vi "Adaptive graph scaling.vi"(7 "Reset buffer":bool, 8 "error in":errorcluster, 9 "Buffer length (points)":i32=10, 10 "Graph data":dbl[](array[numeric]), 11 "GraphChart":refnum<vi>) -> (0 "error out":errorcluster)   [LabVIEW 2017]
uses:
  <userlib>/_MGI/Numeric/Rounding/MGI Round to Decimal Place Enum.ctl
  <vilib>/Analysis/baseanly.llb/Mean (DBL).vi
  <userlib>/_MGI/Application Control/MGI Change Detector/MGI Change Detector (T).vi
  <vilib>/Analysis/NI_AALBase.lvlib
panel:
  # "Use the \"To more generic\" function outside this VI to\nallow using this VI with any type of graph."
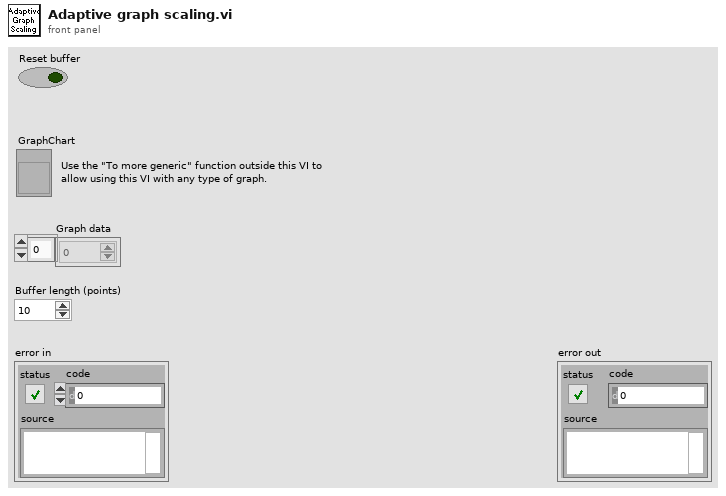
[diagram p1: front panel]
types:
  T1 = typedef "MGI Round to Decimal Place Enum.ctl" = enum16{"Round Nearest", "Round +Inf", "Round -Inf"}
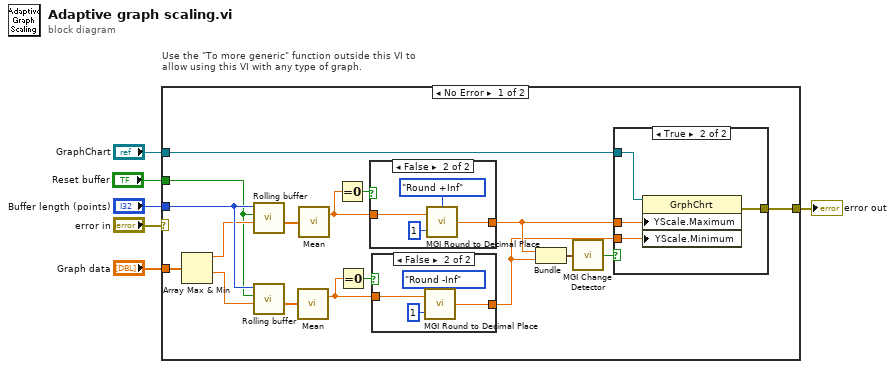
[diagram p0: block diagram]
diagram:
  # "Use the \"To more generic\" function outside this VI to\nallow using this VI with any type of graph."
  n1 = case shown="No Error" "error in" {
    selector: "error in" -> [_ w38]
    tunnel: "Buffer length (points)" -> [w23 _]
    tunnel: "Graph data" -> [w20 _]
    tunnel: "GraphChart" -> [w19 _]
    tunnel: [w8 w38] -> w2
    tunnel: "Reset buffer" -> [w7 _]
    frame No Error {
      n2 = Array Max & Min(array=w20) -> (max value=w22:dbl, min value=w21:dbl)  [unwired: 2 out]
      n3 = call "Rolling buffer.vi"("Value in"=w22, "Reset buffer"=w7, "Buffer length (points)"=w23) -> ("Rolling buffer"=w14:dbl[])  [unwired: 8 in]
      n4 = call "Rolling buffer.vi"("Value in"=w21, "Reset buffer"=w7, "Buffer length (points)"=w23) -> ("Rolling buffer"=w13:dbl[])  [unwired: 8 in]
      n5 = call-poly <vilib>:"Mean.vi"("X"=w13) -> ("mean"=w16:dbl)  [unwired: 1 out]
      n6 = call-poly <vilib>:"Mean.vi"("X"=w14) -> ("mean"=w18:dbl)  [unwired: 1 out]
      n7 = Equal To 0?(x=w18) -> (x = 0?=w17:bool)
      n8 = Equal To 0?(x=w16) -> (x = 0?=w15:bool)
      n9 = case shown="False" w17 {
        tunnel: w18 -> [w33 w35]
        tunnel: [w33 w34] -> w12
        frame True {
        }
        frame False {
          n10 = call <userlib>:"MGI Round to Decimal Place.vi"("Round (To Nearest)"=MGI_Round_to_Decimal_Place_Enum."Round +Inf", "Decimal Digits"=1, "Number"=w35) -> ("Rounded"=w34:dbl)
        }
      }
      n11 = case shown="False" w15 {
        tunnel: w16 -> [w28 w31]
        tunnel: [w28 w30] -> w11
        frame True {
        }
        frame False {
          n12 = call <userlib>:"MGI Round to Decimal Place.vi"("Round (To Nearest)"=MGI_Round_to_Decimal_Place_Enum."Round -Inf", "Decimal Digits"=1, "Number"=w31) -> ("Rounded"=w30:dbl)
        }
      }
      n13 = Bundle("Rounded"=w12, "Rounded"=w11) -> (w10:cluster{"Rounded":dbl, "Rounded":dbl})  [unwired: 1 in]
      n14 = call-poly <userlib>:"MGI Change Detector.vi"("Value"=w10) -> ("Changed?"=w9:bool)
      n15 = case shown="True" w9 {
        tunnel: w12 -> [_ w27]
        tunnel: w11 -> [_ w26]
        tunnel: w19 -> [_ w25]
        tunnel: [_ w24] -> w8
        frame False {
        }
        frame True {
          n16 = property on="Property Node" class="GrphChrt"(reference=w25, "YScale.Maximum"=w27, "YScale.Minimum"=w26) -> (error out=w24:errorcluster)  [unwired: 1 in, 1 out]
        }
      }
    }
    frame Error {
    }
  }
  "error out" <- w2
